vi "Read Hardware.vi"(8 "error in":errorcluster, 11 "Sensor & Control in":refnum<class "Sensor & Control.lvclass">) -> (0 "error out":errorcluster, 3 "Sensor & Control out":refnum<class "Sensor & Control.lvclass">)   [LabVIEW 2013, in "Sensor & Control.lvib.lvlib" / "Sensor & Control.lvclass"]
uses:
  Sensor & Control.lvclass
  Sensor & Control.lvclass/Sensor & Control.ctl
  Read VISA.vi
  Read Value.vi
  PluginInterface/PluginInterface.lvlibp/PluginInterfaceClass/Read Name.vi
  PluginInterface/PluginInterface.lvlibp/PluginInterfaceClass/Read DVR.vi
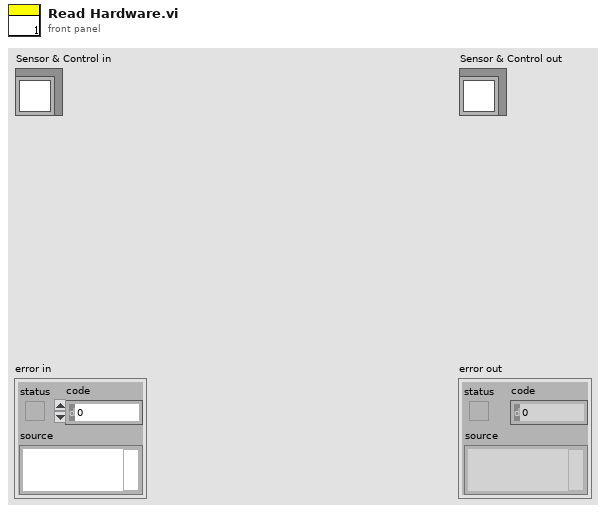
[diagram p1: front panel]
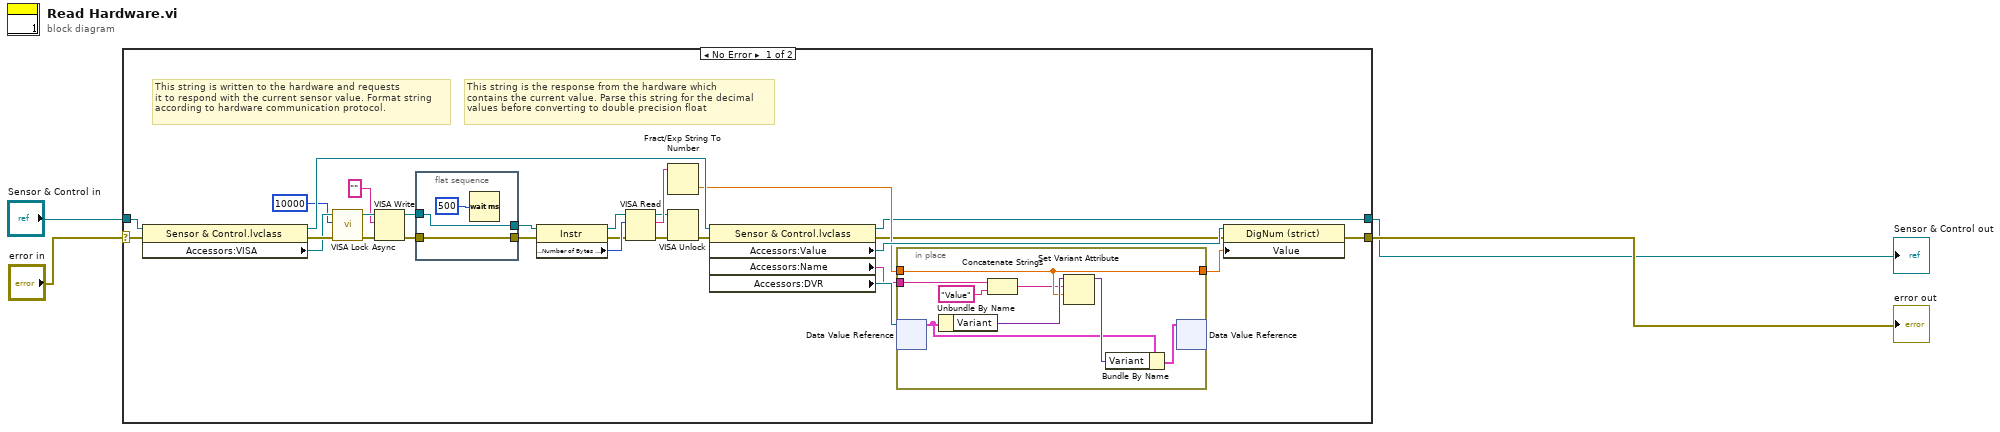
[diagram p0: block diagram]
diagram:
  n1 = case shown="No Error" "error in" {
    selector: "error in" -> [w31 w45]
    tunnel: [w23 w45] -> w3
    tunnel: [w6 w44] -> w1
    tunnel: "Sensor & Control in" -> [w32 w44]
    frame No Error {
      # "This string is the response from the hardware which\ncontains the current value. Parse this string for the decimal \nvalues before converting to double precision float"
      # "This string is written to the hardware and requests\nit to respond with the current sensor value. Format string\naccording to hardware communication protocol."
      n2 = property class="Sensor & Control.lvclass"(reference=w32, error in=w31) -> (reference out=w25:refnum<class "Sensor & Control.lvclass">, error out=w27:errorcluster, "Accessors:VISA"=w26:refnum<visa-resource-name>)
      n3 = call <vilib>:"VISA Lock Async.vi"("error in (no error)"=w27, "timeout (0)"=u32 10000, "VISA resource name"=w26) -> ("error out"=w13:errorcluster, "VISA resource name out"=w14:refnum<visa-resource-name>)  [unwired: 6 in, 1 out]
      n4 = VISA Write(VISA resource name=w14, write buffer="", error in (no error)=w13) -> (VISA resource name out=w22:refnum<visa-resource-name>, error out=w21:errorcluster)  [unwired: 1 out]
      n5 = flat-sequence {
        tunnel: w22 -> [w35]
        tunnel: [w35] -> w16
        tunnel: [w34] -> w20
        tunnel: w21 -> [w34]
        frame #0 {
          n6 = Wait (ms)(milliseconds to wait=u32 500 ("ms before read")) -> ()  [unwired: 1 out]
        }
      }
      n7 = property class="Instr"(reference=w16, error in=w20) -> (reference out=w19:refnum<visa-resource-name>, error out=w17:errorcluster, "Serial Settings:Number of Bytes at Serial Port"=w18:u32)
      n8 = VISA Read(VISA resource name=w19, byte count=w18, error in (no error)=w17) -> (VISA resource name out=w10:refnum<visa-resource-name>, read buffer=w11:string, error out=w9:errorcluster)  [unwired: 1 out]
      n9 = Fract/Exp String To Number(string=w11) -> (number=w24:dbl)  [unwired: 3 in, 1 out]
      n10 = VISA Unlock(8:w9, 11:w10) -> (0:w8:errorcluster)  [unwired: 1 out]
      n11 = property class="Sensor & Control.lvclass"(reference=w25, error in=w8) -> (reference out=w6:refnum<class "Sensor & Control.lvclass">, error out=w5:errorcluster, "Accessors:Value"=w29:refnum<vi>, "Accessors:Name"=w7:string, "Accessors:DVR"=w30:refnum<data-value>)
      n12 = in-place {
        in-place-border: w24 -> [w39]
        in-place-border: [w39] -> w28
        in-place-border: w7 -> [w37]
        n13 = in-place-dvr #1(w30) -> (w40:cluster{"Array":string[], "Variant":variant})  [unwired: 1 out]
        n14 = Unbundle By Name(w40) -> ("Variant"=w42:variant)
        n15 = Concatenate Strings(w37, "Value") -> (w36:string)
        n16 = Set Variant Attribute(Variant=w42, name=w36, value=w39) -> (Variant out=w41:variant)  [unwired: 1 in, 2 out]
        n17 = Bundle By Name(cluster=w40, "Variant"=w41) -> (w43:cluster{"Array":string[], "Variant":variant})
        n18 = in-place-dvr #1(w43) -> ()  [unwired: 2 out]
      }
      n19 = property class="DigNum (strict)"(reference=w29, error in=w5, "Value"=w28) -> (error out=w23:errorcluster)  [unwired: 1 out]
    }
    frame Error {
    }
  }
  "error out" <- w3
  "Sensor & Control out" <- w1
